vi "Init Device.vi"(7 "Layout Ref":refnum<vi>, 8 "error in (no error)":errorcluster, 10 "Chan# Array":i32[](array[numeric]), 11 "Master Device in":refnum<class "Master Device.lvclass">) -> (0 "error out":errorcluster, 3 "Master Device out":refnum<class "Master Device.lvclass">)   [LabVIEW 2013, in "Master Device.lvclass"]
doc: "Initialize the correct columns and their default appearance.\nUse the front panel to change default appearance of the device in the Add/Manage devices.\n\nOpen a specific device implementation for details."
uses:
  Master Device.lvclass
  Device/Device.lvclass
panel:
  # "Open a specific devices override of this VI for implementation."
  # "THIS VI IS NOT USED FOR MASTER DEVICES!!! \n\nProgram initialization instructions using Init Master.vi"
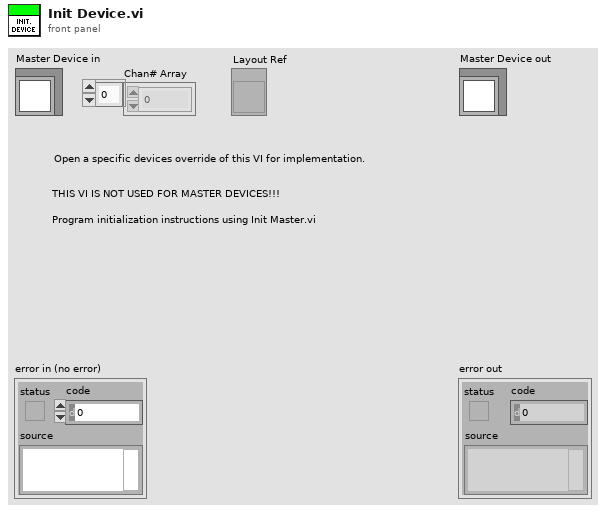
[diagram p1: front panel]
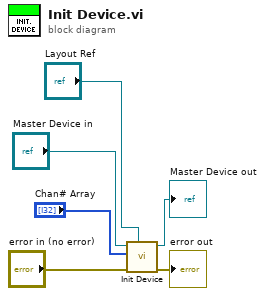
[diagram p0: block diagram]
diagram:
  n1 = call-parent "Init Device.vi"("Layout Ref"="Layout Ref", "error in (no error)"="error in (no error)", "Chan# Array"="Chan# Array", "Device in"="Master Device in") -> ("error out"=→"error out":errorcluster, "Device out"=→"Master Device out":refnum<class "Master Device.lvclass">)  [unwired: 6 in]
